vi "合格状态.vi"(7 "枚举":enum16{"Read", "Write"}(ring), 10 "工位":enum16{"工位一", "工位二"}(ring), 11 "Status_Write":i16) -> (3 "Status_Read":i16)   [LabVIEW 2020]
uses:
  Libraries/S7/S7.lvlib
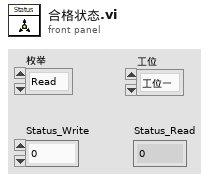
[diagram p1: front panel]
types:
  T1 = typedef "S7.lvlib/Read_Data (Reply Payload)--cluster.ctl" = cluster{"读取成功":bool, "数据":u32[], "Read_Data_error":errorcluster}
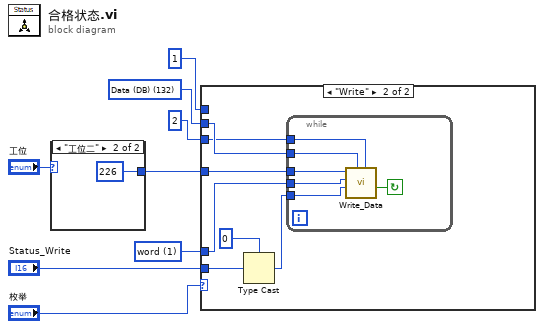
[diagram p0: block diagram]
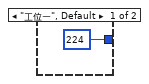
[diagram p2: hidden frame]
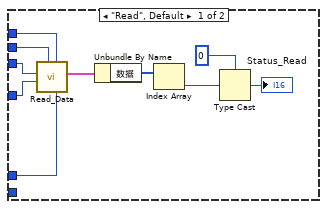
[diagram p3: hidden frame]
diagram:
  w4 = u16 1 items=["byte", "word", "Dword"] ("数据类型")
  w5 = u8 132 items=["I/O (P)"=128, "Input (I)"=129, "Output (Q)"=130, "Bit Memory (M)"=131, "Data (DB)"=132, "Instance Data (DI)"=133, "Local Data (L)"=134, "Predecessor Local Data (VL)"=135] ("寄存器类型")
  n1 = case shown="\"工位二\"" "工位" {
    tunnel: [u32 224 ("起始地址") u32 226 ("起始地址")] -> w1
    frame "工位一", Default {
    }
    frame "工位二" {
    }
  }
  n2 = case shown="\"Write\"" "枚举" {
    tunnel: u16 2 ("DB #") -> [w20 w22]
    tunnel: w1 -> [w16 w21]
    tunnel: w5 -> [w15 w24]
    tunnel: u16 1 ("读取长度") -> [w14 _]
    tunnel: w4 -> [w13 w23]
    tunnel: "Status_Write" -> [_ w25]
    frame "Read", Default {
      n3 = call "Read_Data.vi"("数据类型"=w13, "读取长度"=w14, "寄存器类型"=w15, "起始地址"=w16, "DB #"=w20) -> ("Reply Payload"=w19:T1)  [unwired: 4 in, 2 out]
      n4 = Unbundle By Name(w19) -> ("数据"=w18:u32[])
      n5 = Index Array(array=w18) -> (element=w12:u32)  [unwired: 1 in]
      n6 = Type Cast(type=0, x=w12) -> (*(type *) &x=→"Status_Read":i32)
    }
    frame "Write" {
      n7 = Type Cast(type=u16 0, x=w25) -> (*(type *) &x=w26:u16)
      n8 = while {
        tunnel: w26 -> [w33]
        tunnel: w24 -> [w32]
        tunnel: w23 -> [w31]
        tunnel: w22 -> [w30]
        tunnel: w21 -> [w29]
        stop <- w28 continue-if-true
        n9 = call "Write_Data.vi"("DB #"=w30, "寄存器类型"=w32, "写入数据"=w33, "数据类型"=w31, "写入地址"=w29) -> ("timed out?"=w28:bool)  [unwired: 4 in, 2 out]
      }
    }
  }
